vi "deg_to_rad.vi"(1 "Degrees":dbl) -> (0 "Radians":dbl)   [LabVIEW 2011]
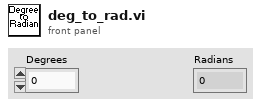
[diagram p1: front panel]
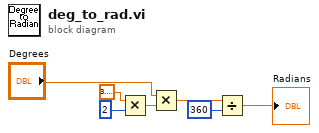
[diagram p0: block diagram]
diagram:
  n1 = Multiply(x=3.141592653589793, y=2) -> (x*y=w3:dbl)
  n2 = Multiply(x="Degrees", y=w3) -> (x*y=w4:dbl)
  n3 = Divide(x=w4, y=360) -> (x/y=→"Radians":dbl)
